vi "Create Plugin Subpanel Events.vi"(8 "error in (no error)":errorcluster) -> (0 "error out":errorcluster, 3 "Plugin Subpanel Events":T1)   [LabVIEW 2021, in "CIF_UI.lvclass"]
uses:
  CIF_UI.lvclass
  Typedef/Plugin Subpanel Events.ctl
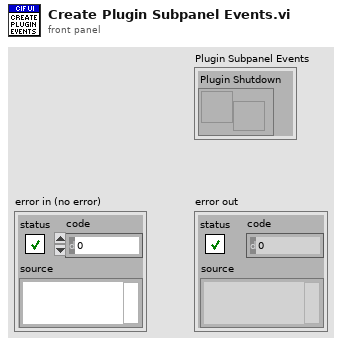
[diagram p1: front panel]
types:
  T1 = typedef "CIF_UI.lvclass/Plugin Subpanel Events.ctl" = cluster{"Plugin Shutdown":refnum<user-event>}
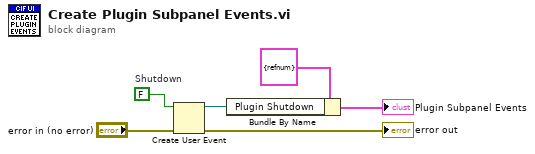
[diagram p0: block diagram]
diagram:
  w6 = FALSE  # Shutdown
  n1 = Create User Event(user event datatype=w6, error in="error in (no error)") -> (user event=w2:refnum<user-event>, error out=→"error out":errorcluster)
  n2 = Bundle By Name(cluster=T1 {"Plugin Shutdown"=refnum} ("Plugin Subpanel Events"), "Plugin Shutdown"=w2) -> (→"Plugin Subpanel Events":T1)
